vi "Update Display.vi"(8 "error in (no error)":errorcluster, 9 "Active Pixels":cluster{"Column":u8, "Row":u8, "Color":u32}[](array[cluster]), 10 "Board State":u32[][](array[numeric]), 11 "Hardware Screen Interface in":refnum<class "Hardware Screen Interface.lvclass">) -> (0 "error out":errorcluster, 3 "Hardware Screen Interface out":refnum<class "Hardware Screen Interface.lvclass">)   [LabVIEW 2017, in "Hardware Screen Interface.lvlib" / "Hardware Screen Interface.lvclass"]
uses:
  Hardware Screen Interface.lvclass
  Screen Interface/Screen Interface/Screen Interface.lvclass
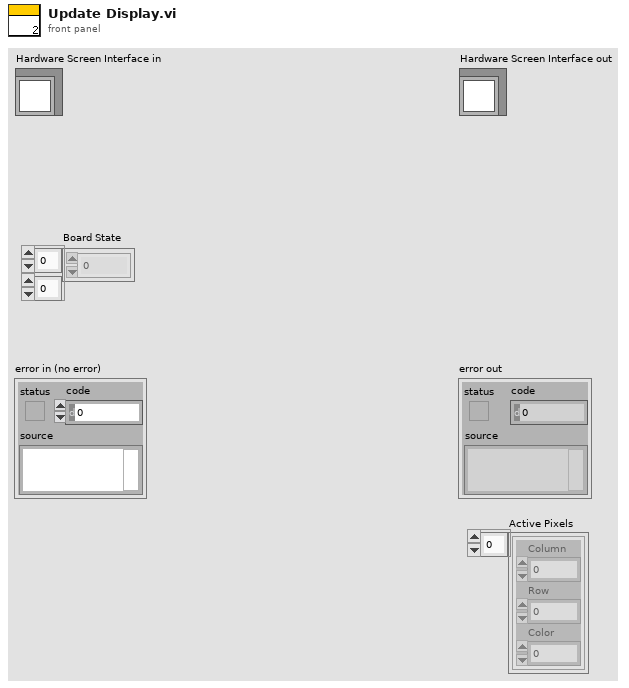
[diagram p1: front panel]
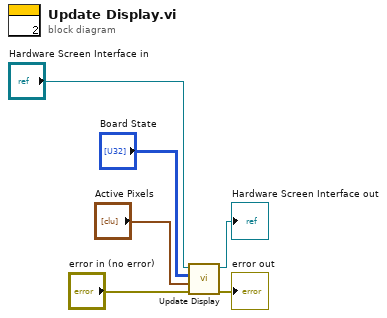
[diagram p0: block diagram]
diagram:
  n1 = call-parent "Update Display.vi"("error in (no error)"="error in (no error)", "Active Pixels"="Active Pixels", "Board State"="Board State", "Screen Interface in"="Hardware Screen Interface in") -> ("error out"=→"error out":errorcluster, "Screen Interface out"=→"Hardware Screen Interface out":refnum<class "Hardware Screen Interface.lvclass">)  [unwired: 6 in]
